vi "Read Pin Map.vi"(8 "error in (no error)":errorcluster, 11 "I-O in":refnum<class "I-O.lvclass">) -> (0 "error out":errorcluster, 2 "Pin Map 2":T1={"Region Valves"=[49, 52, 0, 0], "Extra Valves"=[[[0.0, 48.0, 0.0, 0.0, 0.0]]], "Tool Primary Valve"=51, "Tool Secondary Valve"=50, "Region Sensors"=[37, 41, 37], "Extra Sensors"=[[[36.0, 37.0, 0.0, 0.0]]], "Tool Primary Sensor"=39.0, "Tool Secondary Sensor"=38.0, "Compression Sensor"=31.0, "5V"=50, "Dispenser Sensor"=0.0}, 3 "I-O out":refnum<class "I-O.lvclass">)   [LabVIEW 2018, in "I-O.lvclass"]
uses:
  I-O.lvclass
  Pin Map.ctl
  I-O.lvclass/I-O.ctl
panel:
  out "Pin Map":T1={"Region Valves"=[49, 52, 0, 0], "Extra Valves"=[[[0.0, 48.0, 0.0, 0.0, 0.0]]], "Tool Primary Valve"=51, "Tool Secondary Valve"=50, "Region Sensors"=[37, 41, 37], "Extra Sensors"=[[[36.0, 37.0, 0.0, 0.0]]], "Tool Primary Sensor"=39.0, "Tool Secondary Sensor"=38.0, "Compression Sensor"=31.0, "5V"=50, "Dispenser Sensor"=0.0}
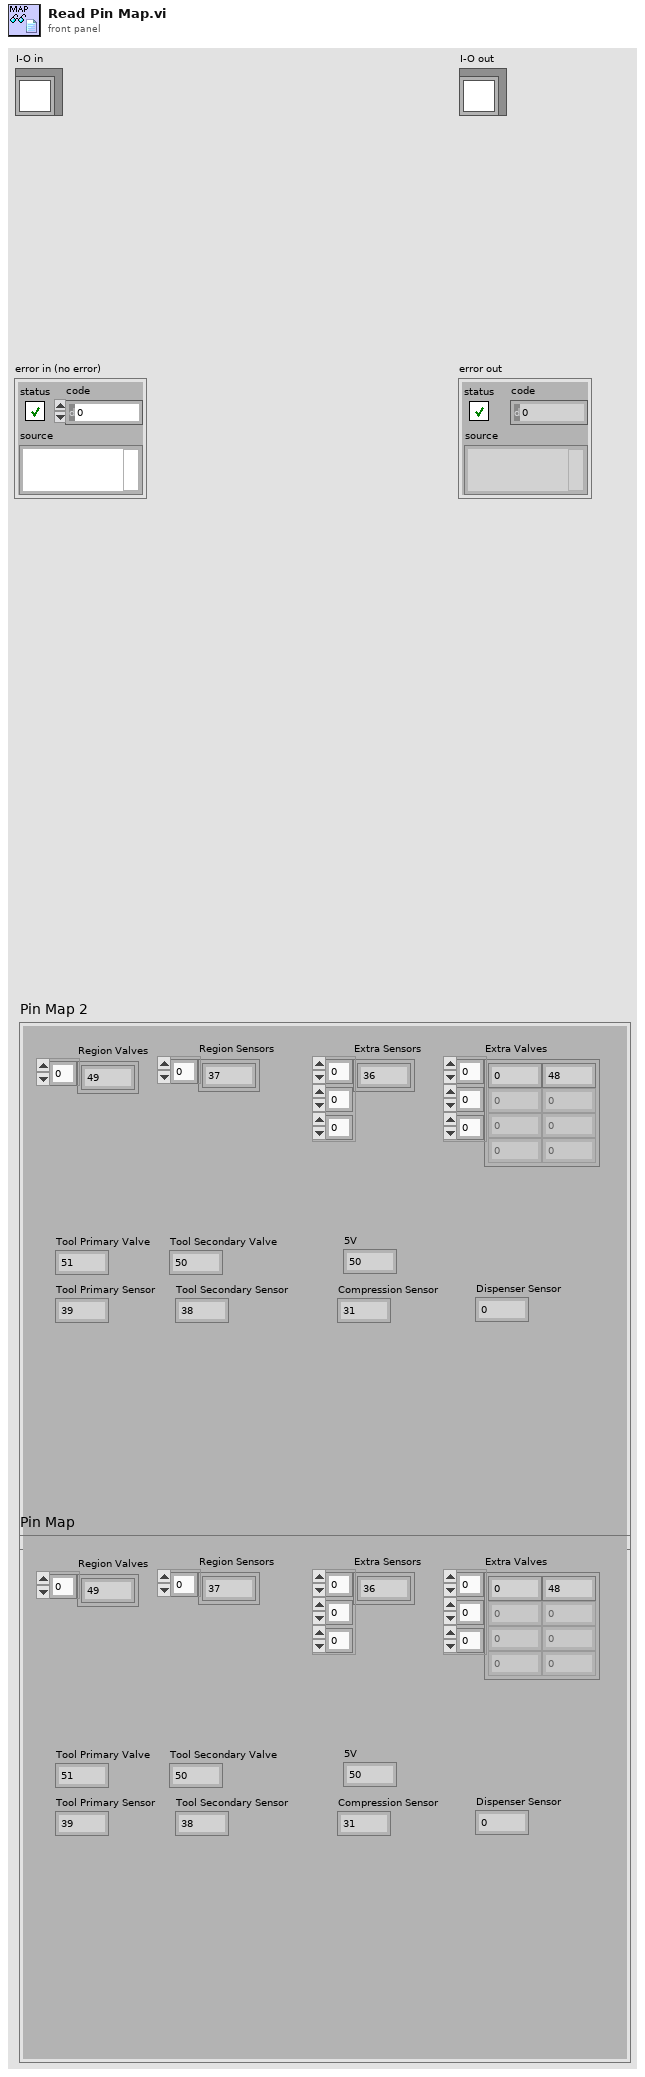
[diagram p1: front panel]
types:
  T1 = typedef "I-O.lvclass/Pin Map.ctl" = cluster{"Region Valves":i32[], "Extra Valves":dbl[][][], "Tool Primary Valve":i32, "Tool Secondary Valve":i32, "Region Sensors":i32[], "Extra Sensors":dbl[][][], "Tool Primary Sensor":dbl, "Tool Secondary Sensor":dbl, "Compression Sensor":dbl, "5V":i32, "Dispenser Sensor":dbl}
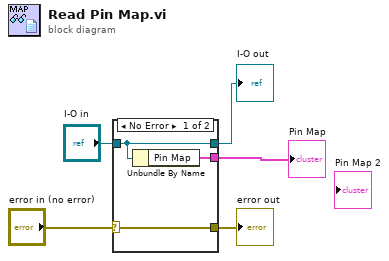
[diagram p0: block diagram]
diagram:
  n1 = case shown="No Error" "error in (no error)" {
    selector: "error in (no error)" -> [w8 w9]
    tunnel: [w8 w9] -> w4
    tunnel: [w7 w10] -> w2
    tunnel: "I-O in" -> [w7 w10]
    tunnel: [w6 _] -> w1
    frame No Error {
      n2 = Unbundle By Name(w7) -> ("Pin Map"=w6:T1)
    }
    frame Error {
    }
  }
  "error out" <- w4
  "I-O out" <- w2
  "Pin Map" <- w1
